vi "sensor touch.vi"() -> ()   [LabVIEW 2016]
uses:
  <vilib>/LabVIEW Interface for Arduino/Type Defs/Board Type.ctl
  <vilib>/LabVIEW Interface for Arduino/Type Defs/Connection Type.ctl
  <vilib>/LabVIEW Interface for Arduino/Type Defs/Pin Mode.ctl
  <vilib>/LabVIEW Interface for Arduino/LabVIEW Interface for Arduino.lvlib
panel:
  in  "?":bool
  out "Boolean":bool
  out "Meter":dbl(knob) scale=0.0..10.0
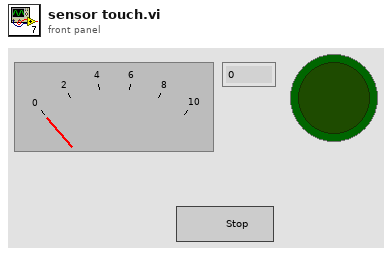
[diagram p1: front panel]
types:
  T1 = typedef "LabVIEW Interface for Arduino.lvlib/Pin Mode.ctl" = enum8{"Input", "Output"}
  T2 = typedef "LabVIEW Interface for Arduino.lvlib/Connection Type.ctl" = enum8{"USB / Serial", "XBEE", "BlueSmirf (Bluetooth)"}
  T3 = typedef "LabVIEW Interface for Arduino.lvlib/Board Type.ctl" = enum16{"Uno", "Dimuelanove w/Atmega 328", "Mega 2560"}
  T4 = typedef "LabVIEW Interface for Arduino.lvlib/Arduino Resource.ctl" = cluster{"VISA resource":refnum<visa-resource-name>, "Board Type":T3, "Connection Type":enum8{"USB / Serial"}, "Bytes Per Packet (15)":u8}
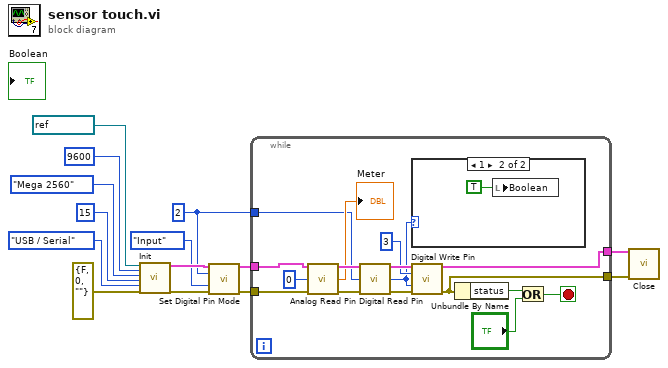
[diagram p0: block diagram]
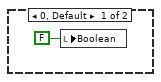
[diagram p2: hidden frame]
diagram:
  w3 = u8 2 ("Digital I/O Pin")
  n1 = call <vilib>:"Init.vi"("VISA resource"=refnum<visa-resource-name> "COM6", "Baud Rate (115200)"=u32 9600, "Board Type (Uno)"=Board_Type."Mega 2560", "Bytes Per Packet (15)"=u32 15, "Connection Type (USB/Serial)"=Connection_Type."USB / Serial", "error in"=errorcluster {"status"=FALSE, "code"=0, "source"=""}) -> ("Arduino Resource"=w8:T4, "error out"=w7:errorcluster)  [unwired: 12 in]
  n2 = call <vilib>:"Set Digital Pin Mode.vi"("Arduino Resource"=w8, "Digital I/O Pin"=w3, "Pin Mode (Input)"=Pin_Mode."Input", "error in"=w7) -> ("Arduino Resource"=w5:T4, "error out"=w4:errorcluster)  [unwired: 10 in]
  n3 = while {
    tunnel: w5 -> [w30]
    tunnel: w4 -> [w29]
    tunnel: w3 -> [w24]
    tunnel: [w19] -> w2
    tunnel: [w18] -> w1
    stop <- w15 stop-if-true
    n4 = call <vilib>:"Analog Read Pin.vi"("Arduino Resource"=w30, "Analog Input Pin (0)"=u8 0, "error in"=w29) -> ("Arduino Resource"=w27:T4, "Voltage"=→"Meter":dbl, "error out"=w26:errorcluster)  [unwired: 10 in]
    n5 = call <vilib>:"Digital Read Pin.vi"("Arduino Resource"=w27, "Digital I/O Pin (0)"=w24, "error in"=w26) -> ("Arduino Resource"=w23:T4, "Value"=w20:u8, "error out"=w22:errorcluster)  [unwired: 10 in]
    n6 = case shown="1" w20 {
      frame 0, Default {
        n7 = local write "Boolean"(FALSE ("Boolean")) -> ()
      }
      frame 1 {
        n8 = local write "Boolean"(TRUE ("Boolean")) -> ()
      }
    }
    n9 = call <vilib>:"Digital Write Pin.vi"("Arduino Resource"=w23, "Digital I/O Pin (0)"=u8 3, "Value (0)"=w20, "error in"=w22) -> ("Arduino Resource"=w19:T4, "error out"=w18:errorcluster)  [unwired: 10 in]
    n10 = Unbundle By Name(w18) -> ("status"=w17:bool)
    n11 = Or(x=w17, y="?") -> (x .or. y?=w15:bool)
  }
  n12 = call <vilib>:"Close.vi"("Arduino Resource"=w2, "error in"=w1) -> ()  [unwired: 13 in, 1 out]
